vi "Reading buffer basetimestamp.vi"(8 "错误输入（无错误）":errorcluster, 10 "仪器型号":string, 11 "VISA资源名称":refnum<visa-resource-name>) -> (0 "错误输出":errorcluster, 2 "时间标识":timestamp, 3 "VISA资源名称输出":refnum<visa-resource-name>)   [LabVIEW 2020]
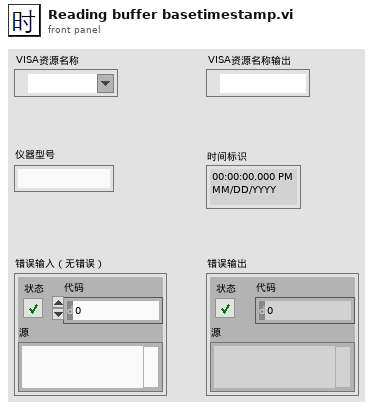
[diagram p1: front panel]
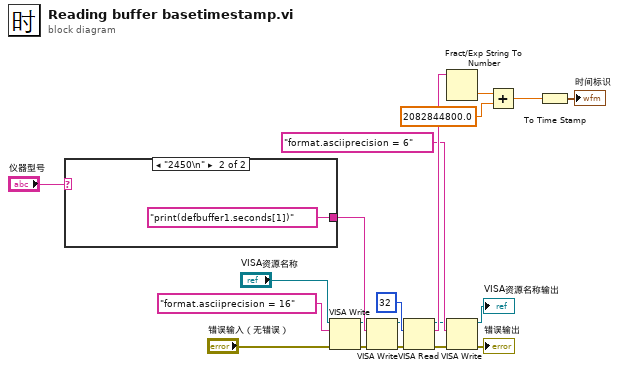
[diagram p0: block diagram]
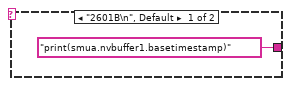
[diagram p2: hidden frame]
diagram:
  n1 = case shown="\"2450\\n\"" "仪器型号" {
    tunnel: ["print(smua.nvbuffer1.basetimestamp)" ("格式字符串") "print(defbuffer1.seconds[1])" ("格式字符串")] -> w8
    frame "2601B\n", Default {
    }
    frame "2450\n" {
    }
  }
  n2 = VISA Write(VISA resource name="VISA资源名称", write buffer="format.asciiprecision = 16" ("格式字符串"), error in (no error)="错误输入（无错误）") -> (VISA resource name out=w3:refnum<visa-resource-name>, error out=w2:errorcluster)  [unwired: 1 out]
  n3 = VISA Write(VISA resource name=w3, write buffer=w8, error in (no error)=w2) -> (VISA resource name out=w12:refnum<visa-resource-name>, error out=w11:errorcluster)  [unwired: 1 out]
  n4 = VISA Read(VISA resource name=w12, byte count=u32 32 ("字节总数"), error in (no error)=w11) -> (VISA resource name out=w10:refnum<visa-resource-name>, read buffer=w18:string, error out=w9:errorcluster)  [unwired: 1 out]
  n5 = Fract/Exp String To Number(string=w18) -> (number=w16:dbl)  [unwired: 3 in, 1 out]
  n6 = VISA Write(VISA resource name=w10, write buffer="format.asciiprecision = 6" ("格式字符串"), error in (no error)=w9) -> (VISA resource name out=→"VISA资源名称输出":refnum<visa-resource-name>, error out=→"错误输出":errorcluster)  [unwired: 1 out]
  n7 = Add(x=w16, y=2082844800.0 ("x-y")) -> (x+y=w15:dbl)
  n8 = To Time Stamp(1:w15) -> (0:→"时间标识":timestamp)
